vi "Get Picture.vi"(8 "error in (no error)":errorcluster, 11 "Circuit Board in":refnum<class "Circuit Board.lvclass">) -> (0 "error out":errorcluster, 2 "Picture":picture, 3 "Circuit Board out":refnum<class "Circuit Board.lvclass">)   [LabVIEW 2020, in "Circuit Board.lvclass"]
uses:
  Circuit Board.lvclass
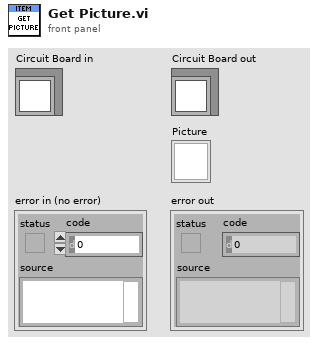
[diagram p1: front panel]
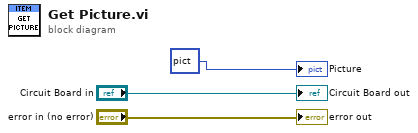
[diagram p0: block diagram]
diagram:
  "error out" <- "error in (no error)"
  "Circuit Board out" <- "Circuit Board in"
  "Picture" <- picture bytes[3230] ("new picture")
